vi "Trigger Pulse Width Query.vi"(8 "error in":errorcluster, 11 "Instrument Handle In":i32) -> (0 "error out":errorcluster, 1 "Level":dbl, 2 "Source":i32, 3 "Instrument Handle Out":i32, 4 "Type":i32 caption="Mode", 5 "Upper Limit":dbl, 6 "Lower Limit":dbl)   [LabVIEW 8.6, in "ZTScopeM.lvlib"]
doc: "Query the pulse-width triggering configuration."
uses:
  ZTScopeM.lvlib
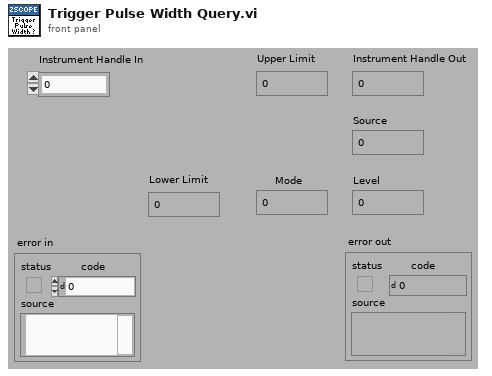
[diagram p1: front panel]
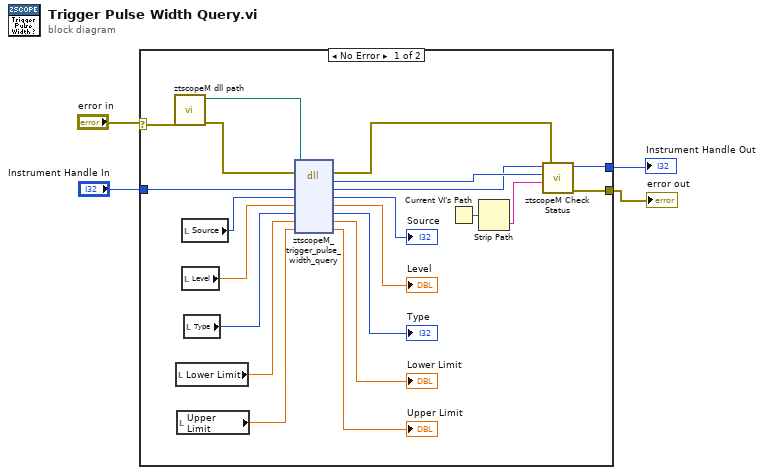
[diagram p0: block diagram]
diagram:
  n1 = case shown="No Error" "error in" {
    selector: "error in" -> [w8 w27]
    tunnel: [w9 w27] -> w1
    tunnel: "Instrument Handle In" -> [w25 w26]
    tunnel: [w10 w26] -> w3
    frame #0 {
      n2 = call "ztscopeM dll path.vi"("error in (no error)"=w8) -> ("error out"=w6:errorcluster, "<instrument>.dll path"=w7:path)  [unwired: 9 in]
      n3 = local read "Lower Limit"() -> (w18:dbl)
      n4 = local read "Upper Limit"() -> (w16:dbl)
      n5 = local read "Source"() -> (w24:i32)
      n6 = local read "Level"() -> (w22:dbl)
      n7 = local read "Type"() -> (w20:i32)
      n8 = dll-call lib="C:/Program Files (x86)/National Instruments/LabVIEW 2013/instr.lib/ztscopem/ztscopeM.dll" fn="ztscopeM_trigger_pulse_width_query"(path in=w7, error in=w6, "instrumentHandle"=w25, "source"=w24, "level"=w22, "mode"=w20, "lowerLimit"=w18, "upperLimit"=w16) -> (error out=w5:errorcluster, w12:i32, "instrumentHandle"=w11:i32, "source"=→"Source":i32, "level"=→"Level":dbl, "mode"=→"Type":i32, "lowerLimit"=→"Lower Limit":dbl, "upperLimit"=→"Upper Limit":dbl)  [unwired: 1 in, 1 out]
      n9 = Current VI's Path() -> (path=w14:path)
      n10 = Strip Path(path=w14) -> (name=w13:string)  [unwired: 1 out]
      n11 = call "ztscopeM Check Status.vi"("error in"=w5, "name of VI"=w13, "status (return code)"=w12, "instrument handle in"=w11) -> ("error out"=w9:errorcluster, "instrument handle out"=w10:i32)  [unwired: 2 in]
    }
    frame #1 {
    }
  }
  "Instrument Handle Out" <- w3
  "error out" <- w1
